vi "SetChanSel.vi"(8 "读取通道选择":T1={"CH 0"=TRUE, "CH 1"=TRUE, "CH 2"=TRUE, "CH 3"=TRUE, "CH 4"=TRUE, "CH 5"=TRUE, "CH 6"=TRUE, "CH 7"=TRUE, "CH 8"=FALSE, "CH 9"=FALSE, "CH 10"=FALSE, "CH 11"=FALSE, "CH 12"=FALSE, "CH 13"=FALSE, "CH 14"=FALSE, "CH 15"=FALSE}, 11 "错误输入":errorcluster) -> (3 "错误输出":errorcluster)   [LabVIEW 2016]
uses:
  PLC-Lab/lib/gusb.dll
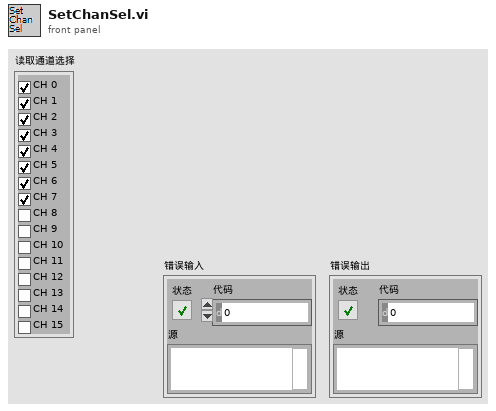
[diagram p1: front panel]
types:
  T1 = cluster{"CH 0":bool, "CH 1":bool, "CH 2":bool, "CH 3":bool, "CH 4":bool, "CH 5":bool, "CH 6":bool, "CH 7":bool, "CH 8":bool, "CH 9":bool, "CH 10":bool, "CH 11":bool, "CH 12":bool, "CH 13":bool, "CH 14":bool, "CH 15":bool}
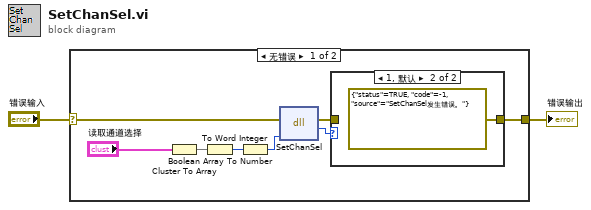
[diagram p0: block diagram]
diagram:
  n1 = case shown="无错误" "错误输入" {
    selector: "错误输入" -> [w4 w13]
    tunnel: [w3 w13] -> w1
    frame No Error {
      n2 = Cluster To Array(cluster="读取通道选择") -> (array=w8:bool[])
      n3 = Boolean Array To Number(Boolean array=w8) -> (number=w10:u32)
      n4 = To Word Integer(number=w10) -> (16bit integer=w9:i16)
      n5 = dll-call lib="E:/Camproject/2018/2018.1Labview/PLC-Lab/lib/gusb.dll" fn="SetChanSel"(error in=w4, "ChanSel"=w9) -> (error out=w5:errorcluster, "Status"=w6:i32)  [unwired: 3 in, 1 out]
      n6 = case shown="1, 默认" w6 {
        tunnel: w5 -> [w11 _]
        tunnel: [w11 errorcluster {"status"=TRUE, "code"=-1, "source"="SetChanSel发生错误。"} ("错误常量")] -> w3
        frame 0 {
        }
        frame 1, Default {
        }
      }
    }
    frame Error {
    }
  }
  "错误输出" <- w1
